vi "KMAX_Spectrometer_driver.vi"(8 "error in":errorcluster, 9 "IntegrationTime (ms)":dbl=5.0 min=5.0 max=1000.0 step=1.0, 10 "New Image":T2, 11 "Camera Name":T1) -> (0 "error out":errorcluster, 1 "Integration Time Output (ms)":dbl, 2 "Image Out":T2, 3 "Session Out":T1, 4 "Wavelengths (nm)":dbl[](array[numeric]), 6 "Intensity":sgl[](array[numeric]))   [LabVIEW 2023]
uses:
  <vilib>/vision/driver/IMAQdx.llb/IMAQdx Attribute Type.ctl
  <vilib>/vision/Image Controls.llb/IMAQ Image.ctl
  <vilib>/userDefined/High Color/IMAQdx.ctl
  <vilib>/vision/driver/IMAQdx.llb/IMAQdx Buffer Number Mode.ctl
  <vilib>/vision/driver/NI_Vision_Acquisition_Software.lvlib
  <vilib>/vision/NI_Vision_Development_Module.lvlib
  <resource>/objmgr/imaqdx.rc
  <resource>/objmgr/IMAQImage.rc
panel:
  out "coerced(x)":dbl
  out "Image":T2(plugin-control)
  out "Line Information 2":T3 {"Standard Deviation" format="%#.2f"; "Mean" format="%#.2f"}
  in  "Row Amount":dbl=5.0
  out "Pixel location vs intensity":sgl[](graph)
  out "Saturated?":bool
  out "Attribute Information Array":T5(array[cluster])
  out "Spectrometer":cluster{dbl[], sgl[]}(graph)
  # "Outputs"
  # "Inputs"
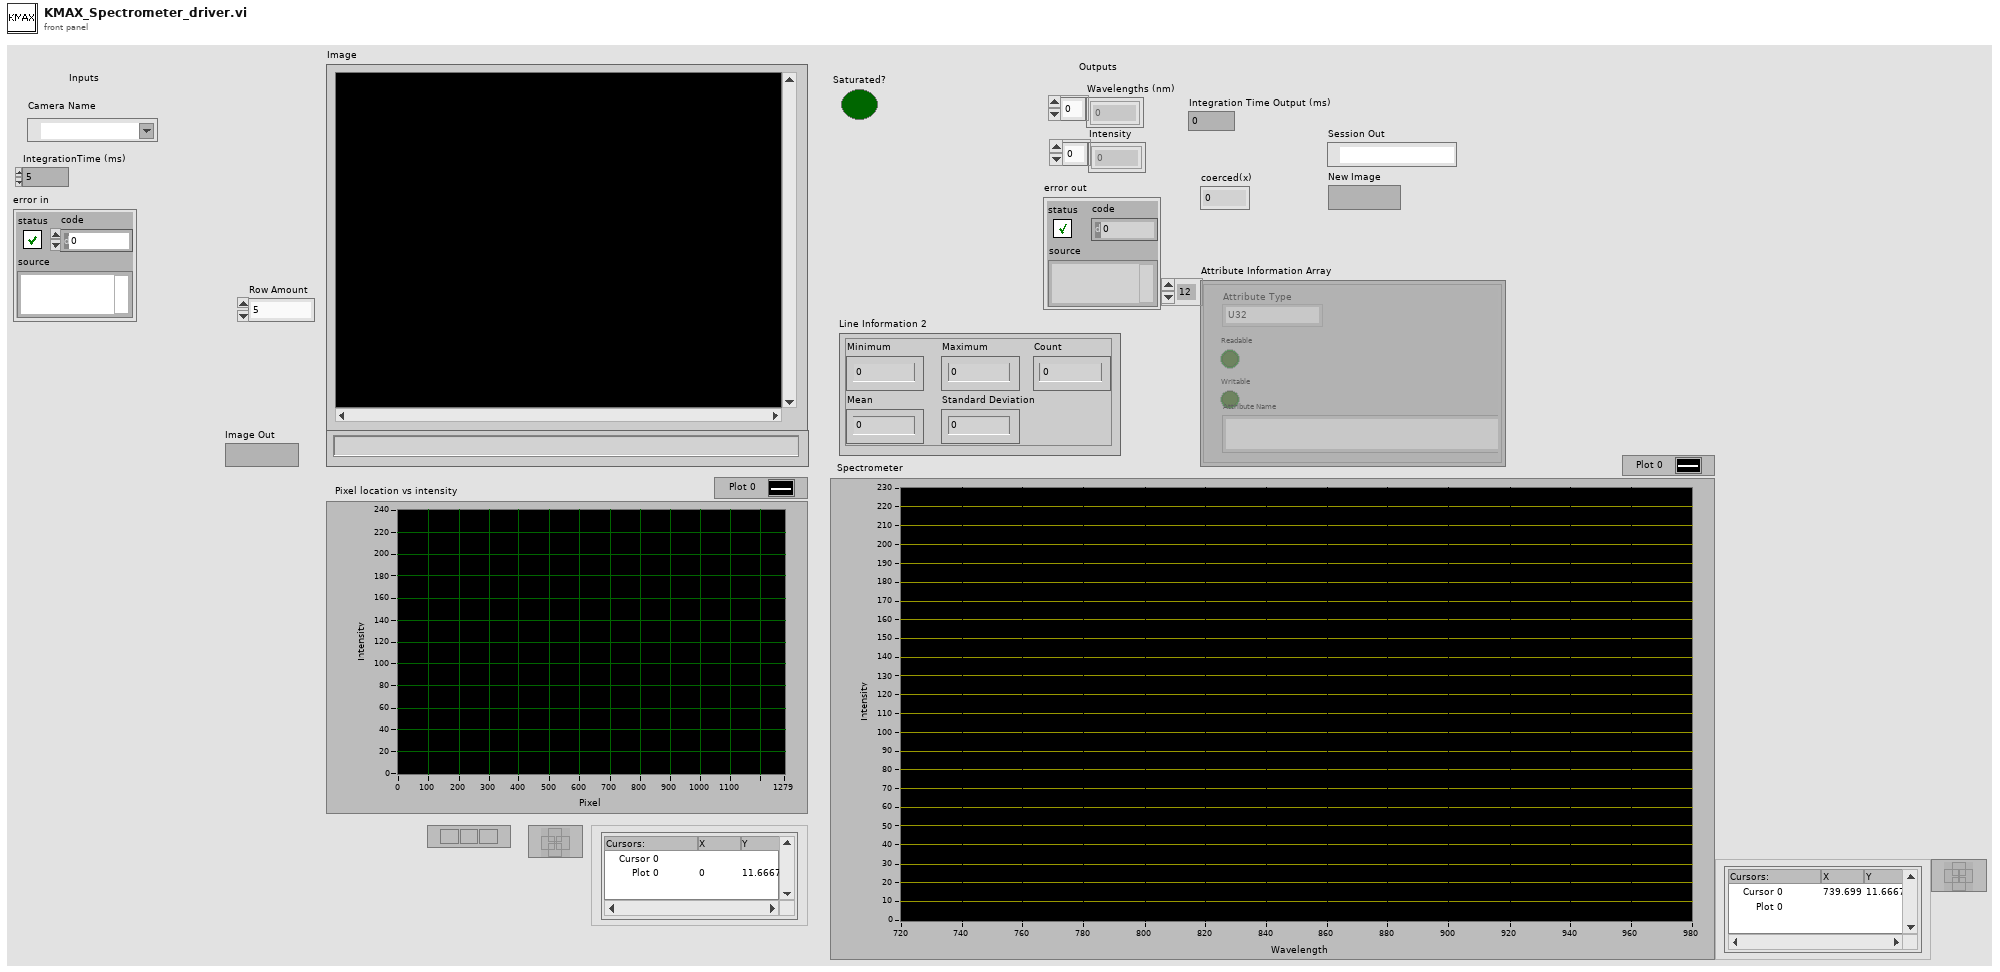
[diagram p1: front panel]
types:
  T1 = typedef "IMAQdx.ctl" = refnum<k21>
  T2 = typedef "IMAQ Image.ctl" = refnum<image>
  T3 = cluster{"Minimum":sgl, "Maximum":sgl, "Mean":sgl, "Standard Deviation":sgl, "Count":i32}
  T4 = typedef "NI_Vision_Acquisition_Software.lvlib/IMAQdx Attribute Type.ctl" = enum32{"U32", "I64", "DBL", "String", "Enum", "Bool", "Command"}
  T5 = cluster{"Attribute Type":T4, "Readable":bool, "Writable":bool, "Attribute Name":string}[]
  T6 = typedef "NI_Vision_Acquisition_Software.lvlib/IMAQdx Buffer Number Mode.ctl" = enum32{"Next", "Last", "Buffer Number", "Every", "Last New"}
  T7 = cluster{"Min":sgl, "Max":sgl, "Mean":sgl, "Std Dev":sgl, "Count":i32}
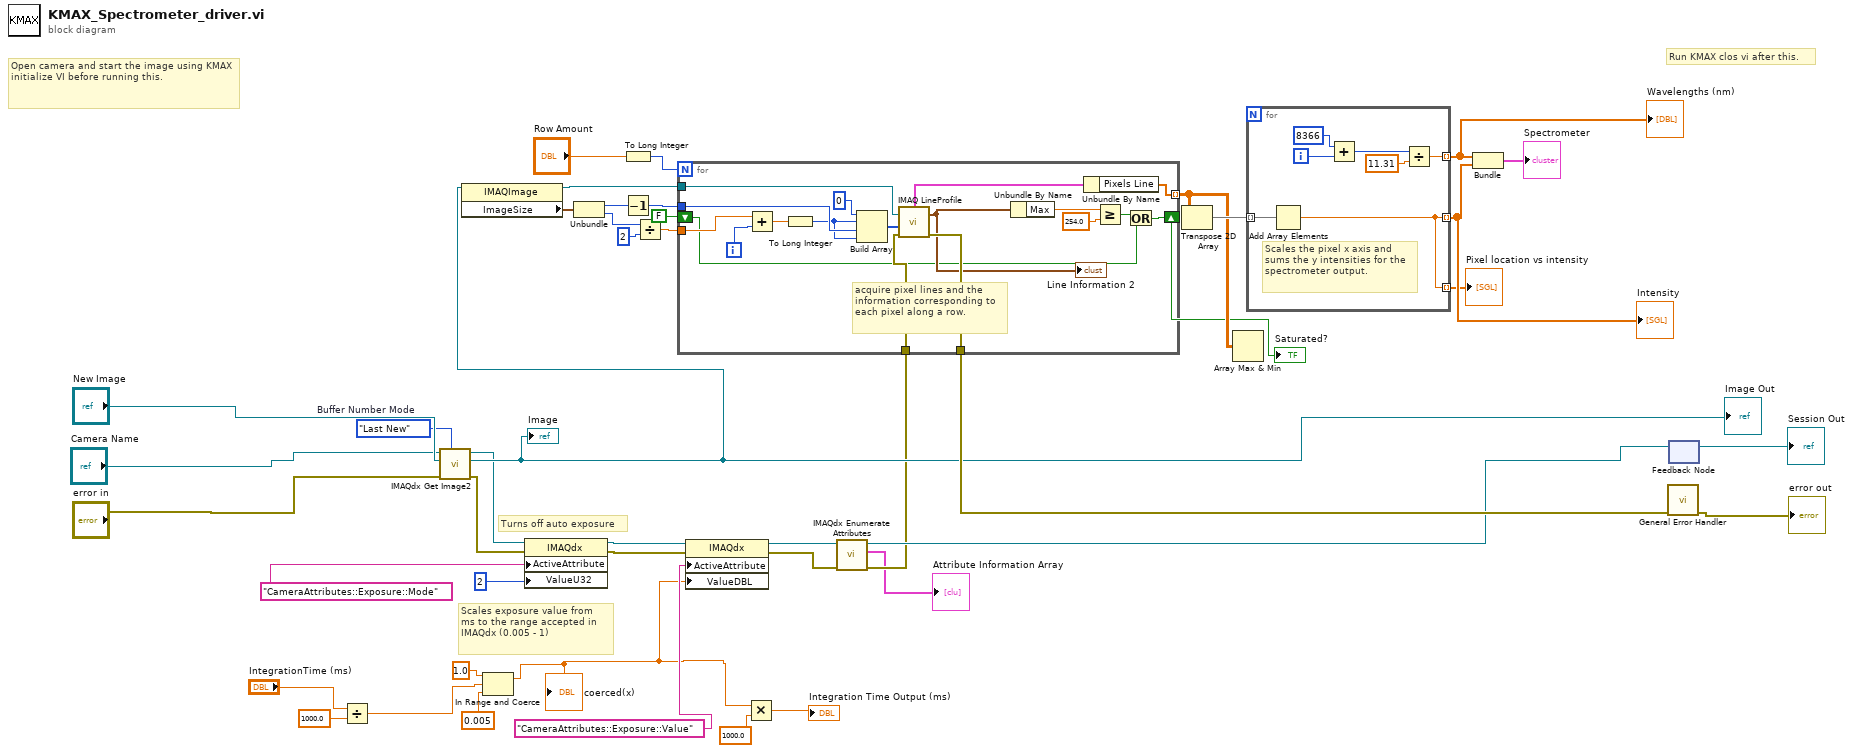
[diagram p0: block diagram]
diagram:
  w35 = IMAQdx_Buffer_Number_Mode."Last New"  # Buffer Number Mode
  # "Scales exposure value from\nms to the range accepted in\nIMAQdx (0.005 - 1)"
  # "Turns off auto exposure"
  # "Run KMAX clos vi after this."
  # "Open camera and start the image using KMAX initialize VI before running this."
  n1 = Divide(x="IntegrationTime (ms)", y=1000.0) -> (x/y=w4:dbl)
  n2 = call <vilib>:"IMAQdx Get Image2.vi"("Buffer Number Mode (Next)"=w35, "error in"="error in", "Image In"="New Image", "Session In"="Camera Name") -> ("error out"=w19:errorcluster, "Image Out"=w36:T2, "Session Out"=w18:T1)  [unwired: 4 in, 1 out]
  "Image Out" <- w36
  "Image" <- w36
  n3 = property class="IMAQImage"(reference=w36) -> (reference out=w9:T2, "ImageSize"=w29:cluster{"x":i32, "y":i32})  [unwired: 1 in, 1 out]
  n4 = In Range and Coerce(upper limit=1.0, x=w4, lower limit=0.005) -> (coerced(x)=w1:dbl)  [unwired: 1 out]
  "coerced(x)" <- w1
  n5 = property class="IMAQdx"(reference=w18, error in=w19, "ActiveAttribute"="CameraAttributes::Exposure::Mode", "ValueU32"=u32 2) -> (reference out=w14:T1, error out=w15:errorcluster)
  n6 = Unbundle(w29) -> ("x"=w34:i32, "y"=w32:i32)
  n7 = To Long Integer(number="Row Amount") -> (32bit integer=w27:i32)
  n8 = Decrement(x=w34) -> (x-1=w33:i32)
  n9 = Divide(x=w32, y=2) -> (x/y=w30:dbl)
  n10 = property class="IMAQdx"(reference=w14, error in=w15, "ActiveAttribute"="CameraAttributes::Exposure::Value", "ValueDBL"=w1) -> (reference out=w12:T1, error out=w13:errorcluster)
  n11 = Multiply(x=w1, y=1000.0) -> (x*y=→"Integration Time Output (ms)":dbl)
  n12 = call <vilib>:"IMAQdx Enumerate Attributes.vi"("error in"=w13, "Session In"=w12) -> ("error out"=w21:errorcluster, "Attribute Information Array"=→"Attribute Information Array":T5, "Session Out"=w38:T1)  [unwired: 7 in]
  n13 = for {
    N: w27 -> [_]
    tunnel: w33 -> [w62]
    tunnel: w30 -> [w61]
    tunnel: w21 -> [w57]
    tunnel: [w56] -> w40
    tunnel: [w53] -> w24 mode=indexing
    shift-right: [w47] -> w22
    shift-left: FALSE -> [w48]
    tunnel: w9 -> [w46]
    i -> [w60]
    # "acquire pixel lines and the information corresponding to each pixel along a row."
    n14 = Add(x=w61, y=w60) -> (x+y=w59:dbl)
    n15 = To Long Integer(number=w59) -> (32bit integer=w58:i32)
    n16 = Build Array(0, w58, w62, w58) -> (w55:i32[])
    n17 = call "IMAQ LineProfile"("error in (no error)"=w57, "Line Coordinates"=w55, "Image"=w46) -> ("error out"=w56:errorcluster, "Line Graph"=w54:cluster{"x0":sgl, "dx":sgl, "Pixels Line":sgl[]}, "Line Information"=w52:T7)  [unwired: 2 in, 1 out]
    "Line Information 2" <- w52
    n18 = Unbundle By Name(w52) -> ("Max"=w51:sgl)
    n19 = Unbundle By Name(w54) -> ("Pixels Line"=w53:sgl[])
    n20 = Greater Or Equal?(x=w51, y=sgl 254.0) -> (x >= y?=w49:bool)
    n21 = Or(x=w49, y=w48) -> (x .or. y?=w47:bool)
  }
  "Saturated?" <- w22
  n22 = Transpose 2D Array(2D array=w24) -> (transposed array=w26:sgl[][])
  n23 = Array Max & Min(array=w24) -> ()  [unwired: 4 out]
  n24 = for {
    tunnel: w26 -> [w70] mode=indexing
    tunnel: [w64] -> w25 mode=indexing
    tunnel: [w65] -> w45 mode=indexing
    tunnel: [w64] -> w43 mode=indexing
    i -> [w66]
    # "Scales the pixel x axis and sums the y intensities for the spectrometer output."
    n25 = Add Array Elements(numeric array=w70) -> (sum=w64:sgl)
    n26 = Add(x=8366, y=w66) -> (x+y=w68:i32)
    n27 = Divide(x=w68, y=11.31) -> (x/y=w65:dbl)
  }
  "Wavelengths (nm)" <- w45
  "Intensity" <- w43
  "Pixel location vs intensity" <- w25
  n28 = Bundle(w45, w43) -> (→"Spectrometer":cluster{dbl[], sgl[]})  [unwired: 1 in]
  n29 = call <vilib>:"General Error Handler.vi"("error in (no error)"=w40) -> ("error out"=→"error out":errorcluster)  [unwired: 2 in, 12 out]
  n30 = feedback-in #1(w38) -> ()
  n31 = feedback #1() -> (→"Session Out":T1)  [unwired: 1 in]
